vi "Autonomous Independent.vi"   [LabVIEW 2018]
doc: "This VI is called when autonomous begins, and will automatically be terminated when autonomous ends. You can carry out timed or sensor driven robot movement independently without needing to return to the caller."
uses:
  <vilib>/Rock Robotics/WPI/Solenoid/WPI_SolenoidValue.ctl
  <vilib>/Rock Robotics/Network Tables/NT Write Numeric Array.vi
  Robot Global Data.vi
  <vilib>/Rock Robotics/WPI/Solenoid/WPI_SolenoidSetEnum.vi
  <vilib>/Rock Robotics/Network Tables/NT Read String.vi
  <vilib>/Rock Robotics/WPI/RobotDrive/WPI_RobotDriveArcadeDrive_Standard(NoSaturation).vi
panel:
  # "Be sure to right-click and choose Data Operations>>Make Current Value default if you want to save the array values with the VI"
types:
  T1 = typedef "WPI_SolenoidValue.ctl" = enum16{"Off", "On", "Forward", "Reverse"}
  T2 = typedef "WPI_SolenoidDevRef.ctl" = cluster{"DevStatus":errorcluster, "Pneumatics Control Module":u8, "Forward Solenoid Channel":T3, "Reverse Solenoid Channel":T3}
  T3 = typedef "WPI_SolenoidChannel.ctl" = enum8{"Solenoid 0", "Solenoid 1", "Solenoid 2", "Solenoid 3", "Solenoid 4", "Solenoid 5", "Solenoid 6", "Solenoid 7", "Invalid"}
  T4 = typedef "WPI_RobotDriveDevRef.ctl" = cluster{"DevStatus":errorcluster, "Motors[]":T5[], "Square Inputs":bool, "Max Output":dbl}
  T5 = typedef "WPI_MotorControlDeviceRef.ctl" = cluster{"DeviceStatus":errorcluster, "Type":T6, "PWM":cluster{"PWM Channel":T7, "DeadBand":T8}, "CAN":cluster{"Device Number":u8, "SetOutput VI Ref":variant, "GetOutput VI Ref":variant, "Enable VI Ref":variant, "Disable VI Ref":variant, "Data":variant}, "Invert":bool, "DIO PWM":cluster{"PWM \"Enable\" Channel":T7, "DIOChannel":T9, "PWM Rate":dbl}}
  T6 = typedef "WPI_MotorControlType.ctl" = enum16{"PWM", "CAN", "DIO PWM"}
  T7 = typedef "FPGA_DIOPWMChannel.ctl" = enum8{"PWM 0", "PWM 1", "PWM 2", "PWM 3", "PWM 4", "PWM 5", "PWM 6", "PWM 7", "PWM 8", "PWM 9", "PWM MXP 0", "PWM MXP 1", "PWM MXP 2", "PWM MXP 3", "PWM MXP 4", "PWM MXP 5", "PWM MXP 6", "PWM MXP 7", "PWM MXP 8", "PWM MXP 9", "Invalid"}
  T8 = typedef "WPI_PWMDeadband.ctl" = cluster{"Name":string, "maxPositivePwm":i32, "minPositivePwm":i32, "centerPwm":i32, "maxNegativePwm":i32, "minNegativePwm":i32, "angularRange":u16}
  T9 = typedef "FPGA_DIOChannel.ctl" = enum8{"DIO 0", "DIO 1", "DIO 2", "DIO 3", "DIO 4", "DIO 5", "DIO 6", "DIO 7", "DIO 8", "DIO 9", "DIO MXP 0", "DIO MXP 1", "DIO MXP 2", "DIO MXP 3", "DIO MXP 4", "DIO MXP 5", "DIO MXP 6", "DIO MXP 7", "DIO MXP 8", "DIO MXP 9", "DIO MXP 10", "DIO MXP 11", "DIO MXP 12", "DIO MXP 13", "DIO MXP 14", "DIO MXP 15", "SPI Port CS1", "SPI Port CS2", "SPI Port CS3", "SPI Port MISO", "SPI Port MOSI", "Invalid"}
  T10 = typedef "WPI_JoystickDevRef.ctl" = cluster{"Device":T11}
  T11 = typedef "WPI_JoystickDeviceEnum.ctl" = enum16{"USB 0", "USB 1", "USB 2", "USB 3", "USB 4", "USB 5"}
  T12 = typedef "WPI_DriverStationPositionInfo.ctl" = enum16{"1", "2", "3"}
  T13 = typedef "WPI_DriverStationAllianceInfo.ctl" = enum16{"Red", "Blue", "Invalid"}
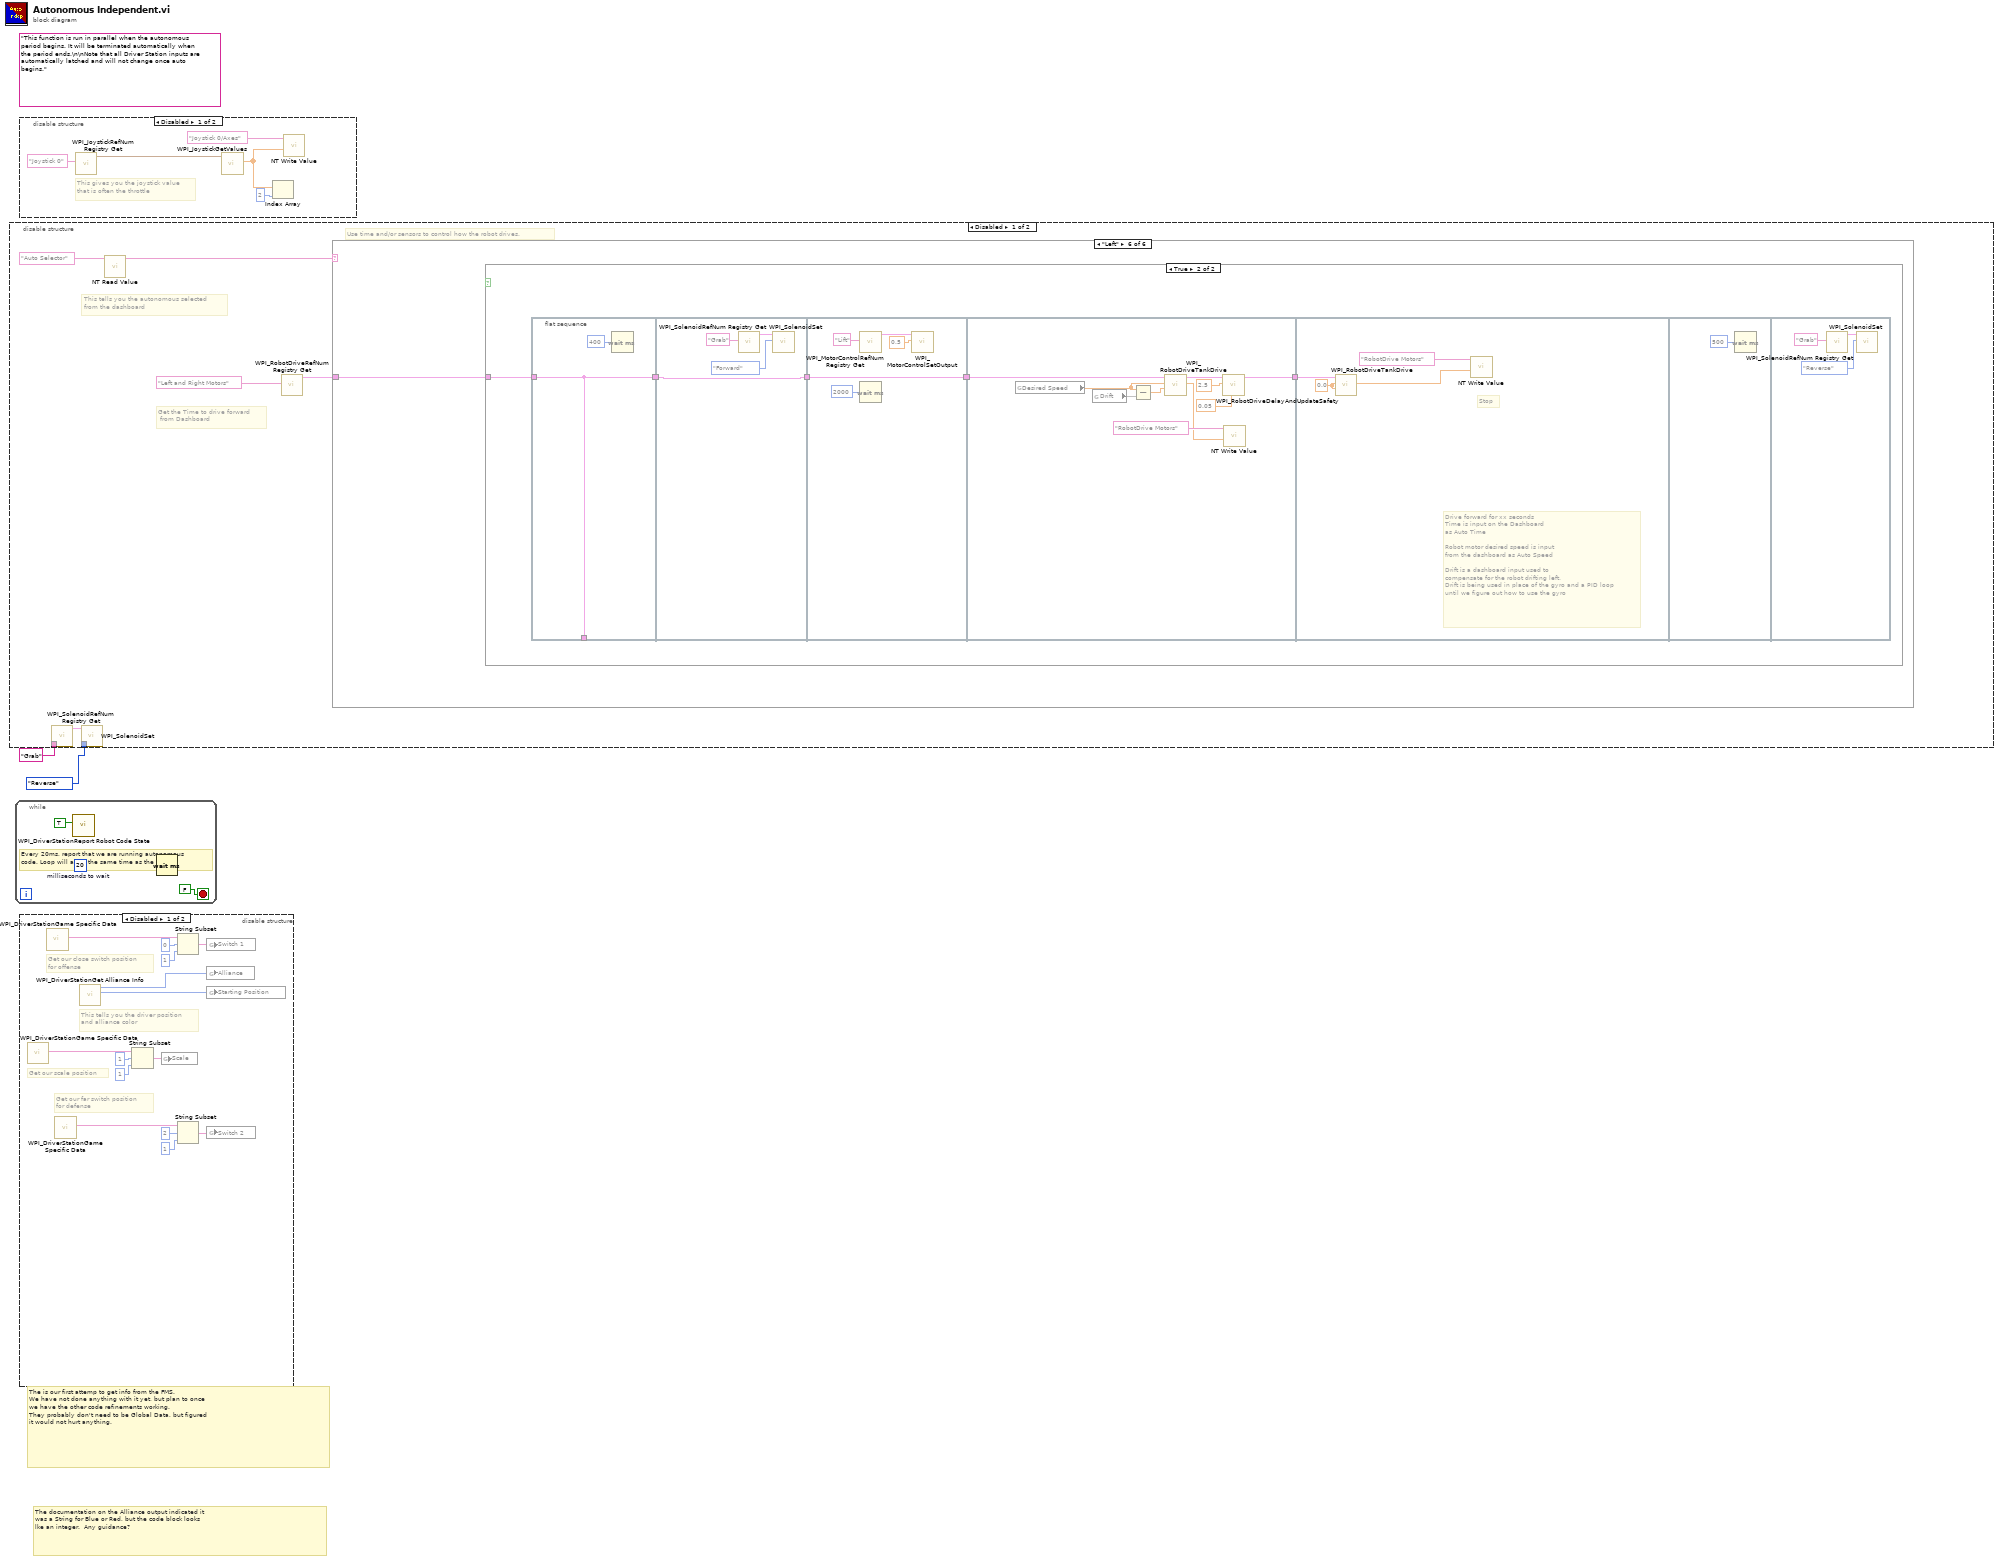
[diagram p0: block diagram]
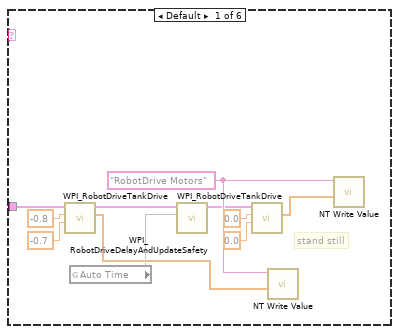
[diagram p2: hidden frame]
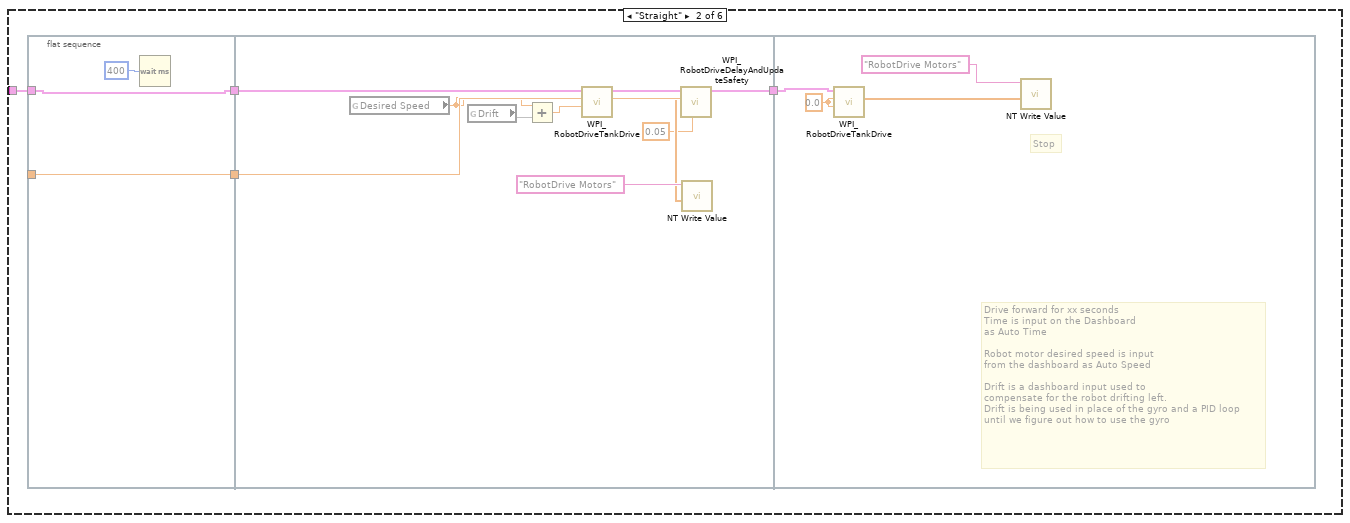
[diagram p3: hidden frame]
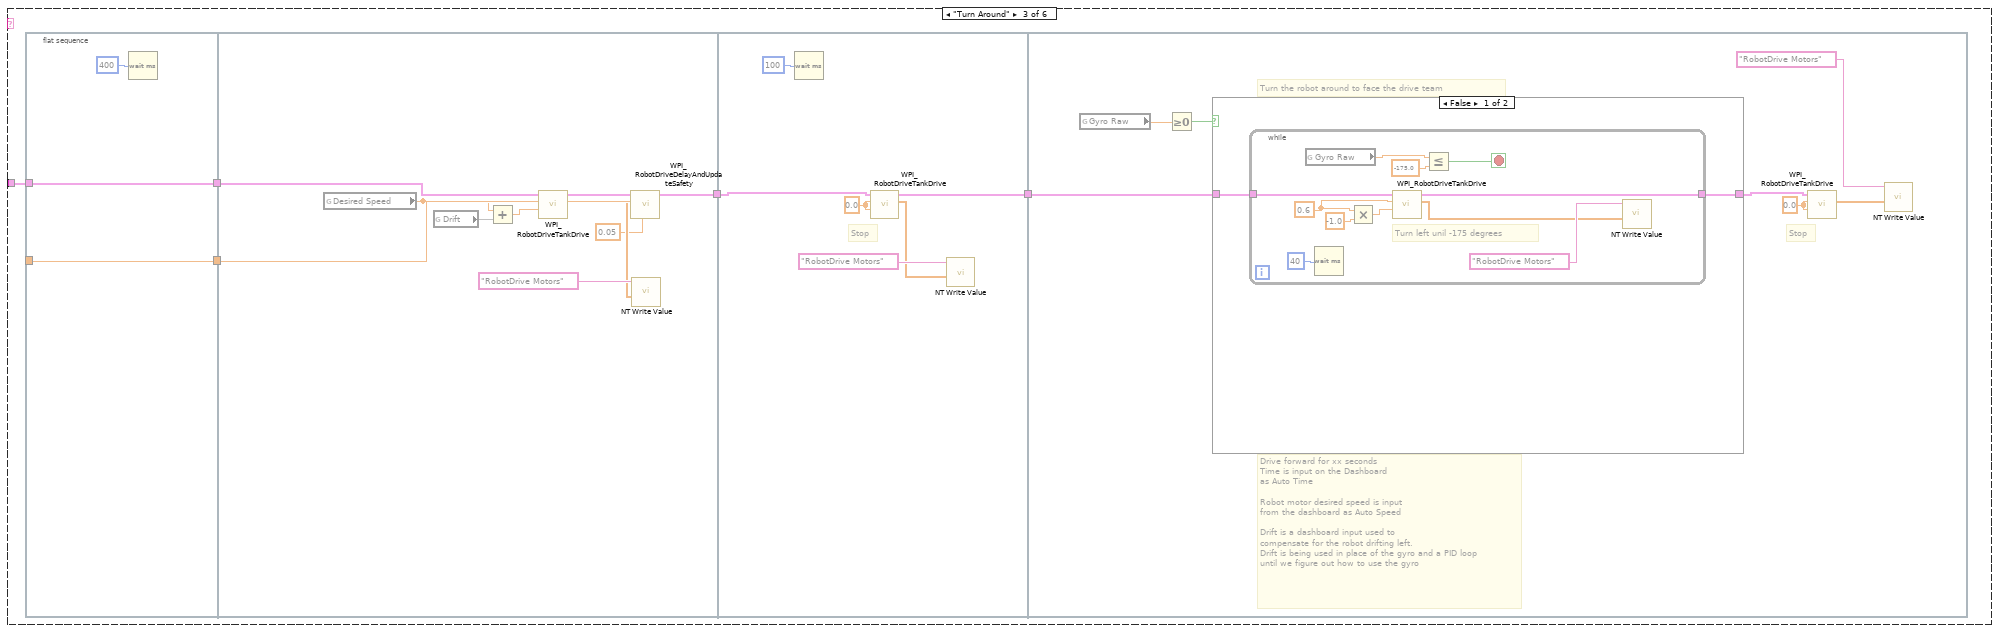
[diagram p4: hidden frame]
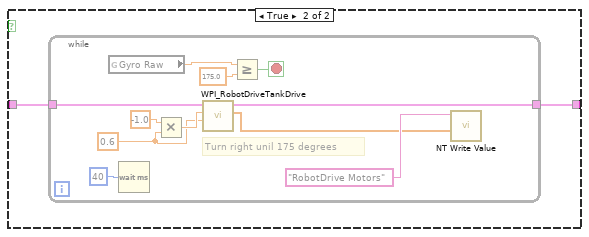
[diagram p5: hidden frame]
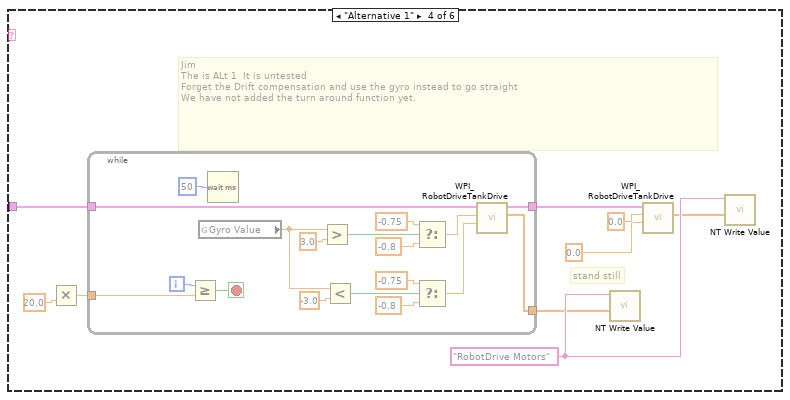
[diagram p6: hidden frame]
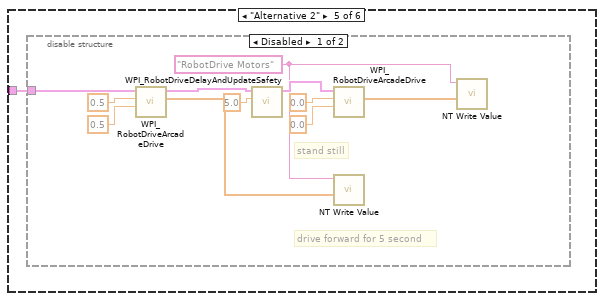
[diagram p7: hidden frame]
diagram:
  (unwired) "This function is run in parallel when the autonomous period begins. It will be terminated automatically when the period ends.\n\nNote that all Driver Station inputs are automatically latched and will not change once auto begins."
  # "The documentation on the Alliance output indicated it\nwas a String for Blue or Red, but the code block looks\nlke an integer.  Any guidance?"
  # "The is our first attemp to get info from the FMS.\nWe have not done anything with it yet, but plan to once\nwe have the other code refinements working.\nThey probably don't need to be Global Data, but figured\nit would not hurt anything."
  n1 = disable-structure shown="Disabled" {
    disable-tunnel: WPI_SolenoidValue."Reverse" ("Value") -> [w5 _]
    disable-tunnel: "Grab" ("refnum name") -> [w4 _]
    frame Disabled {
      # "Get the Time to drive forward\n from Dashboard"
      # "This tells you the autonomous selected\nfrom the dashboard"
      # "Use time and/or sensors to control how the robot drives."
      n2 = call <vilib>:"WPI_SolenoidRefNum Registry Get.vi"("refnum name"=w4) -> ("SolenoidDevRef"=w3:T2)  [unwired: 9 in, 1 out]
      n3 = call-poly <vilib>:"WPI_SolenoidSet.vi"("Value"=w5, "SolenoidDevRef"=w3) -> ()  [unwired: 8 in, 2 out]
      n4 = call-poly <vilib>:"NT Read Value.vi"("Name"="Auto Selector") -> ("String"=w8:string)  [unwired: 9 in, 1 out]
      n5 = call <vilib>:"WPI_RobotDriveRefNum Registry Get.vi"("refnum name"="Left and Right Motors") -> ("RobotDriveDevRef"=w6:T4)  [unwired: 1 in, 9 out]
      n6 = case shown="\"Left\"" w8 {
        tunnel: w6 -> [w19 w24 w46 w99 w127 w139]
        frame Default {
          w20 = "RobotDrive Motors" ("Name")
          # "stand still"
          n7 = call <vilib>:"WPI_RobotDriveTankDrive.vi"("Right axis value"=-0.7 ("X axis value"), "Left axis value"=-0.8, "RobotDriveDevRef"=w19) -> ("Motor Values"=w18:dbl[], "RobotDriveDevRef"=w17:T4)  [unwired: 6 in, 1 out]
          n8 = global read "Robot Global Data.vi" "Auto Time"() -> (w10)
          n9 = call <vilib>:"WPI_RobotDriveDelayAndUpdateSafety.vi"("Delay (s)"=w10, "RobotDriveDevRef"=w17) -> ("RobotDriveDevRef 2"=w16:T4)  [unwired: 8 in, 1 out]
          n10 = call <vilib>:"WPI_RobotDriveTankDrive.vi"("Right axis value"=0.0 ("X axis value"), "Left axis value"=0.0 ("X axis value"), "RobotDriveDevRef"=w16) -> ("Motor Values"=w13:dbl[])  [unwired: 6 in, 2 out]
          n11 = call-poly <vilib>:"NT Write Value.vi"("Numeric Array"=w18, "Name"=w20) -> ()  [unwired: 9 in, 1 out]
          n12 = call-poly <vilib>:"NT Write Value.vi"("Numeric Array"=w13, "Name"=w20) -> ()  [unwired: 9 in, 1 out]
        }
        frame "Straight" {
          n13 = flat-sequence {
            tunnel: _ -> [w26]
            tunnel: w24 -> [w27]
            tunnel: [w27] -> w22
            tunnel: [w26] -> w21
            tunnel: [w30] -> w23
            tunnel: w22 -> [w34]
            tunnel: w21 -> [w33]
            tunnel: w23 -> [w38]
            frame #0 {
              n14 = Wait (ms)(milliseconds to wait=u32 400) -> ()  [unwired: 1 out]
            }
            frame #1 {
              n15 = global read "Robot Global Data.vi" "Desired Speed"() -> (w28:dbl)
              n16 = global read "Robot Global Data.vi" "Drift"() -> (w35)
              n17 = Add(x=w28, y=w35) -> (x+y=w36:dbl)
              n18 = call <vilib>:"WPI_RobotDriveTankDrive.vi"("Right axis value"=w36, "Left axis value"=w28, "RobotDriveDevRef"=w34) -> ("Motor Values"=w31:dbl[], "RobotDriveDevRef"=w37:T4)  [unwired: 6 in, 1 out]
              n19 = call <vilib>:"WPI_RobotDriveDelayAndUpdateSafety.vi"("Feed time (s)"=0.05, "Delay (s)"=w33, "RobotDriveDevRef"=w37) -> ("RobotDriveDevRef 2"=w30:T4)  [unwired: 7 in, 1 out]
              n20 = call-poly <vilib>:"NT Write Value.vi"("Numeric Array"=w31, "Name"="RobotDrive Motors") -> ()  [unwired: 9 in, 1 out]
            }
            frame #2 {
              w41 = 0.0 ("Right axis value")
              # "Drive forward for xx seconds\nTime is input on the Dashboard\nas Auto Time\n\nRobot motor desired speed is input\nfrom the dashboard as Auto Speed\n\nDrift is a dashboard input used to\ncompensate for the robot drifting left.\nDrift is being used in place of the gyro and a PID loop\nuntil we figure out how to use the gyro"
              # "Stop"
              n21 = call <vilib>:"WPI_RobotDriveTankDrive.vi"("Right axis value"=w41, "Left axis value"=w41, "RobotDriveDevRef"=w38) -> ("Motor Values"=w39:dbl[])  [unwired: 6 in, 2 out]
              n22 = call-poly <vilib>:"NT Write Value.vi"("Numeric Array"=w39, "Name"="RobotDrive Motors") -> ()  [unwired: 9 in, 1 out]
            }
          }
        }
        frame "Turn Around" {
          n23 = flat-sequence {
            tunnel: _ -> [w48]
            tunnel: w46 -> [w49]
            tunnel: [w49] -> w43
            tunnel: [w48] -> w42
            tunnel: [w52] -> w45
            tunnel: w43 -> [w56]
            tunnel: w42 -> [w55]
            tunnel: w45 -> [w63]
            tunnel: [w61] -> w44
            tunnel: w44 -> [w66]
            frame #0 {
              n24 = Wait (ms)(milliseconds to wait=u32 400) -> ()  [unwired: 1 out]
            }
            frame #1 {
              n25 = global read "Robot Global Data.vi" "Desired Speed"() -> (w50:dbl)
              n26 = global read "Robot Global Data.vi" "Drift"() -> (w57)
              n27 = Add(x=w50, y=w57) -> (x+y=w58:dbl)
              n28 = call <vilib>:"WPI_RobotDriveTankDrive.vi"("Right axis value"=w58, "Left axis value"=w50, "RobotDriveDevRef"=w56) -> ("Motor Values"=w53:dbl[], "RobotDriveDevRef"=w59:T4)  [unwired: 6 in, 1 out]
              n29 = call <vilib>:"WPI_RobotDriveDelayAndUpdateSafety.vi"("Feed time (s)"=0.05, "Delay (s)"=w55, "RobotDriveDevRef"=w59) -> ("RobotDriveDevRef 2"=w52:T4)  [unwired: 7 in, 1 out]
              n30 = call-poly <vilib>:"NT Write Value.vi"("Numeric Array"=w53, "Name"="RobotDrive Motors") -> ()  [unwired: 9 in, 1 out]
            }
            frame #2 {
              w64 = 0.0 ("Right axis value")
              # "Stop"
              n31 = Wait (ms)(milliseconds to wait=u32 100) -> ()  [unwired: 1 out]
              n32 = call <vilib>:"WPI_RobotDriveTankDrive.vi"("Right axis value"=w64, "Left axis value"=w64, "RobotDriveDevRef"=w63) -> ("Motor Values"=w62:dbl[], "RobotDriveDevRef"=w61:T4)  [unwired: 6 in, 1 out]
              n33 = call-poly <vilib>:"NT Write Value.vi"("Numeric Array"=w62, "Name"="RobotDrive Motors") -> ()  [unwired: 9 in, 1 out]
            }
            frame #3 {
              w72 = 0.0 ("Right axis value")
              # "Turn the robot around to face the drive team"
              # "Stop"
              # "Drive forward for xx seconds\nTime is input on the Dashboard\nas Auto Time\n\nRobot motor desired speed is input\nfrom the dashboard as Auto Speed\n\nDrift is a dashboard input used to\ncompensate for the robot drifting left.\nDrift is being used in place of the gyro and a PID loop\nuntil we figure out how to use the gyro"
              n34 = global read "Robot Global Data.vi" "Gyro Raw"() -> (w67:dbl)
              n35 = Greater Or Equal To 0?(x=w67) -> (x >= 0?=w68:bool)
              n36 = case shown="False" w68 {
                tunnel: [w74 w86] -> w71
                tunnel: w66 -> [w73 w87]
                frame False {
                  n37 = while {
                    tunnel: [w85] -> w74
                    tunnel: w73 -> [w79]
                    stop <- w84 stop-if-true
                    w76 = 0.6 ("Left axis value")
                    # "Turn left unil -175 degrees"
                    n38 = global read "Robot Global Data.vi" "Gyro Raw"() -> (w82:dbl)
                    n39 = Wait (ms)(milliseconds to wait=u32 40) -> ()  [unwired: 1 out]
                    n40 = Multiply(x=w76, y=-1.0) -> (x*y=w78:dbl)
                    n41 = call <vilib>:"WPI_RobotDriveTankDrive.vi"("Right axis value"=w78, "Left axis value"=w76, "RobotDriveDevRef"=w79) -> ("Motor Values"=w80:dbl[], "RobotDriveDevRef"=w85:T4)  [unwired: 6 in, 1 out]
                    n42 = Less Or Equal?(x=w82, y=-175.0) -> (x <= y?=w84:bool)
                    n43 = call-poly <vilib>:"NT Write Value.vi"("Numeric Array"=w80, "Name"="RobotDrive Motors") -> ()  [unwired: 9 in, 1 out]
                  }
                }
                frame True {
                  n44 = while {
                    tunnel: [w98] -> w86
                    tunnel: w87 -> [w92]
                    stop <- w97 stop-if-true
                    w89 = 0.6 ("Left axis value")
                    # "Turn right unil 175 degrees"
                    n45 = global read "Robot Global Data.vi" "Gyro Raw"() -> (w95:dbl)
                    n46 = Wait (ms)(milliseconds to wait=u32 40) -> ()  [unwired: 1 out]
                    n47 = Multiply(x=-1.0, y=w89) -> (x*y=w91:dbl)
                    n48 = call <vilib>:"WPI_RobotDriveTankDrive.vi"("Right axis value"=w89, "Left axis value"=w91, "RobotDriveDevRef"=w92) -> ("Motor Values"=w93:dbl[], "RobotDriveDevRef"=w98:T4)  [unwired: 6 in, 1 out]
                    n49 = Greater Or Equal?(x=w95, y=175.0) -> (x >= y?=w97:bool)
                    n50 = call-poly <vilib>:"NT Write Value.vi"("Numeric Array"=w93, "Name"="RobotDrive Motors") -> ()  [unwired: 9 in, 1 out]
                  }
                }
              }
              n51 = call <vilib>:"WPI_RobotDriveTankDrive.vi"("Right axis value"=w72, "Left axis value"=w72, "RobotDriveDevRef"=w71) -> ("Motor Values"=w69:dbl[])  [unwired: 6 in, 2 out]
              n52 = call-poly <vilib>:"NT Write Value.vi"("Numeric Array"=w69, "Name"="RobotDrive Motors") -> ()  [unwired: 9 in, 1 out]
            }
          }
        }
        frame "Alternative 1" {
          w108 = "RobotDrive Motors" ("Name")
          # "Jim\nThe is ALt 1  It is untested\nForget the Drift compensation and use the gyro instead to go straight\nWe have not added the turn around function yet."
          # "stand still"
          n53 = Multiply(y=20.0) -> (x=w100:dbl, x*y=w101:dbl)
          n54 = while {
            tunnel: [w113] -> w103
            tunnel: [w112] -> w104
            tunnel: w101 -> [w111]
            tunnel: w99 -> [w109]
            i -> [w115]
            stop <- w114 stop-if-true
            n55 = Greater Or Equal?(x=w115, y=w111) -> (x >= y?=w114:bool)
            n56 = global read "Robot Global Data.vi" "Gyro Value"() -> (w110:dbl)
            n57 = Wait (ms)(milliseconds to wait=u32 50) -> ()  [unwired: 1 out]
            n58 = Greater?(x=w110, y=3.0) -> (0:w120:bool)
            n59 = Less?(x=w110, y=-3.0) -> (x < y?=w125:bool)
            n60 = Select(t=-0.75, s=w120, f=-0.8) -> (s? t:f=w117:dbl)
            n61 = Select(t=-0.75, s=w125, f=-0.8) -> (s? t:f=w122:dbl)
            n62 = call <vilib>:"WPI_RobotDriveTankDrive.vi"("Right axis value"=w122, "Left axis value"=w117, "RobotDriveDevRef"=w109) -> ("Motor Values"=w112:dbl[], "RobotDriveDevRef"=w113:T4)  [unwired: 6 in, 1 out]
          }
          n63 = call-poly <vilib>:"NT Write Value.vi"("Numeric Array"=w104, "Name"=w108) -> ()  [unwired: 9 in, 1 out]
          n64 = call <vilib>:"WPI_RobotDriveTankDrive.vi"("Right axis value"=0.0 ("X axis value"), "Left axis value"=0.0 ("X axis value"), "RobotDriveDevRef"=w103) -> ("Motor Values"=w105:dbl[])  [unwired: 6 in, 2 out]
          n65 = call-poly <vilib>:"NT Write Value.vi"("Numeric Array"=w105, "Name"=w108) -> ()  [unwired: 9 in, 1 out]
        }
        frame "Alternative 2" {
          n66 = disable-structure shown="Disabled" {
            disable-tunnel: w127 -> [w128 _]
            frame Disabled {
              w129 = "RobotDrive Motors" ("Name")
              # "stand still"
              # "drive forward for 5 second"
              n67 = call-poly <vilib>:"WPI_RobotDriveArcadeDrive.vi"("Y axis value"=0.5 ("X axis value"), "X axis value"=0.5, "RobotDriveDevRef"=w128) -> ("Motor Values"=w132:dbl[], "RobotDriveDevRef"=w138:T4)  [unwired: 1 in, 6 out]
              n68 = call <vilib>:"WPI_RobotDriveDelayAndUpdateSafety.vi"("Delay (s)"=5.0 ("X axis value"), "RobotDriveDevRef"=w138) -> ("RobotDriveDevRef 2"=w131:T4)  [unwired: 8 in, 1 out]
              n69 = call-poly <vilib>:"WPI_RobotDriveArcadeDrive.vi"("Y axis value"=0.0 ("X axis value"), "X axis value"=0.0, "RobotDriveDevRef"=w131) -> ("Motor Values"=w133:dbl[])  [unwired: 1 in, 7 out]
              n70 = call-poly <vilib>:"NT Write Value.vi"("Numeric Array"=w132, "Name"=w129) -> ()  [unwired: 9 in, 1 out]
              n71 = call-poly <vilib>:"NT Write Value.vi"("Numeric Array"=w133, "Name"=w129) -> ()  [unwired: 9 in, 1 out]
            }
            frame Enabled {
            }
          }
        }
        frame "Left" {
          n72 = case shown="True" {
            selector: _ -> [_ _]
            tunnel: w139 -> [_ w140]
            frame False {
            }
            frame True {
              n73 = flat-sequence {
                tunnel: [w145] -> _
                tunnel: [w145] -> w144
                tunnel: w140 -> [w145]
                tunnel: w144 -> [w150]
                tunnel: [w150] -> w143
                tunnel: w143 -> [w155]
                tunnel: [w155] -> w142
                tunnel: [w159] -> w141
                tunnel: w142 -> [w162]
                tunnel: w141 -> [w166]
                frame #0 {
                  n74 = Wait (ms)(milliseconds to wait=u32 400) -> ()  [unwired: 1 out]
                }
                frame #1 {
                  n75 = call <vilib>:"WPI_SolenoidRefNum Registry Get.vi"("refnum name"="Grab") -> ("SolenoidDevRef"=w148:T2)  [unwired: 9 in, 1 out]
                  n76 = call-poly <vilib>:"WPI_SolenoidSet.vi"("Value"=WPI_SolenoidValue."Forward", "SolenoidDevRef"=w148) -> ()  [unwired: 8 in, 2 out]
                }
                frame #2 {
                  n77 = call <vilib>:"WPI_MotorControlRefNum Registry Get.vi"("refnum name"="Lift") -> ("MotorControlDevRef"=w153:T5)  [unwired: 9 in, 1 out]
                  n78 = Wait (ms)(milliseconds to wait=u32 2000) -> ()  [unwired: 1 out]
                  n79 = call <vilib>:"WPI_MotorControlSetOutput.vi"("Output"=0.5, "MotorControlDevRef"=w153) -> ()  [unwired: 7 in, 3 out]
                }
                frame #3 {
                  n80 = global read "Robot Global Data.vi" "Desired Speed"() -> (w157:dbl)
                  n81 = global read "Robot Global Data.vi" "Drift"() -> (w163)
                  n82 = Subtract(x=w157, y=w163) -> (x-y=w164:dbl)
                  n83 = call <vilib>:"WPI_RobotDriveTankDrive.vi"("Right axis value"=w164, "Left axis value"=w157, "RobotDriveDevRef"=w162) -> ("Motor Values"=w160:dbl[], "RobotDriveDevRef"=w165:T4)  [unwired: 6 in, 1 out]
                  n84 = call <vilib>:"WPI_RobotDriveDelayAndUpdateSafety.vi"("Feed time (s)"=0.05, "Delay (s)"=2.5, "RobotDriveDevRef"=w165) -> ("RobotDriveDevRef 2"=w159:T4)  [unwired: 7 in, 1 out]
                  n85 = call-poly <vilib>:"NT Write Value.vi"("Numeric Array"=w160, "Name"="RobotDrive Motors") -> ()  [unwired: 9 in, 1 out]
                }
                frame #4 {
                  w169 = 0.0 ("Right axis value")
                  # "Drive forward for xx seconds\nTime is input on the Dashboard\nas Auto Time\n\nRobot motor desired speed is input\nfrom the dashboard as Auto Speed\n\nDrift is a dashboard input used to\ncompensate for the robot drifting left.\nDrift is being used in place of the gyro and a PID loop\nuntil we figure out how to use the gyro"
                  # "Stop"
                  n86 = call <vilib>:"WPI_RobotDriveTankDrive.vi"("Right axis value"=w169, "Left axis value"=w169, "RobotDriveDevRef"=w166) -> ("Motor Values"=w167:dbl[])  [unwired: 6 in, 2 out]
                  n87 = call-poly <vilib>:"NT Write Value.vi"("Numeric Array"=w167, "Name"="RobotDrive Motors") -> ()  [unwired: 9 in, 1 out]
                }
                frame #5 {
                  n88 = Wait (ms)(milliseconds to wait=u32 500) -> ()  [unwired: 1 out]
                }
                frame #6 {
                  n89 = call <vilib>:"WPI_SolenoidRefNum Registry Get.vi"("refnum name"="Grab") -> ("SolenoidDevRef"=w172:T2)  [unwired: 9 in, 1 out]
                  n90 = call-poly <vilib>:"WPI_SolenoidSet.vi"("Value"=WPI_SolenoidValue."Reverse", "SolenoidDevRef"=w172) -> ()  [unwired: 8 in, 2 out]
                }
              }
            }
          }
        }
      }
    }
    frame Enabled {
    }
  }
  n91 = while {
    stop <- FALSE stop-if-true
    w174 = u32 20  # milliseconds to wait
    # "Every 20ms, report that we are running autonomous\ncode. Loop will abort the same time as the VI."
    n92 = call <vilib>:"WPI_DriverStationReport Robot Code State.vi"("Autonomous"=TRUE) -> ()  [unwired: 10 in, 1 out]
    n93 = Wait (ms)(milliseconds to wait=w174) -> ()  [unwired: 1 out]
  }
  n94 = disable-structure shown="Disabled" {
    frame Disabled {
      # "This gives you the joystick value\nthat is often the throttle"
      n95 = call <vilib>:"WPI_JoystickRefNum Registry Get.vi"("refnum name"="Joystick 0") -> ("JoystickDevRef"=w180:T10)  [unwired: 1 in, 9 out]
      n96 = call <vilib>:"WPI_JoystickGetValues.vi"("JoystickDevRef"=w180) -> ("Axes"=w178:dbl[])  [unwired: 6 in, 4 out]
      n97 = Index Array(array=w178, index=2) -> ()  [unwired: 1 out]
      n98 = call-poly <vilib>:"NT Write Value.vi"("Numeric Array"=w178, "Name"="Joystick 0/Axes") -> ()  [unwired: 9 in, 1 out]
    }
    frame Enabled {
    }
  }
  n99 = disable-structure shown="Disabled" {
    frame Disabled {
      # "Get our scale position"
      # "Get our far switch position\nfor defense"
      # "Get our close switch position\nfor offense"
      # "This tells you the driver position\nand alliance color"
      n100 = call <vilib>:"WPI_DriverStationGame Specific Data.vi"() -> ("Game Specific Data"=w190:string)  [unwired: 11 in]
      n101 = call <vilib>:"WPI_DriverStationGame Specific Data.vi"() -> ("Game Specific Data"=w195:string)  [unwired: 11 in]
      n102 = call <vilib>:"WPI_DriverStationGame Specific Data.vi"() -> ("Game Specific Data"=w189:string)  [unwired: 11 in]
      n103 = call <vilib>:"WPI_DriverStationGet Alliance Info.vi"() -> ("Position"=w183:T12, "Alliance"=w182:T13)  [unwired: 10 out]
      n104 = String Subset(string=w190, offset (0)=1, length (rest)=1 ("length (rest)")) -> (substring=w185:string)
      n105 = global write "Robot Global Data.vi" "Scale"(w185) -> ()
      n106 = String Subset(string=w195, offset (0)=0, length (rest)=1 ("length (rest)")) -> (substring=w186:string)
      n107 = String Subset(string=w189, offset (0)=2, length (rest)=1 ("length (rest)")) -> (substring=w184:string)
      n108 = global write "Robot Global Data.vi" "Switch 1"(w186) -> ()
      n109 = global write "Robot Global Data.vi" "Alliance"(w182) -> ()
      n110 = global write "Robot Global Data.vi" "Starting Position"(w183) -> ()
      n111 = global write "Robot Global Data.vi" "Switch 2"(w184) -> ()
    }
    frame Enabled {
    }
  }
